vi "oscillograph (2).vi"() -> ()   [LabVIEW 2013]
panel:
  out "Fall time":string
  out "Rise time":string
  out "Period":string
  out "Vrms":string
  out "Vpp":string
  in  "Channels":T1(radio)
  in  "Exit":bool
  out "Waveform Graph":u8[](graph)
  in  "VISA Address":refnum<visa-resource-name>
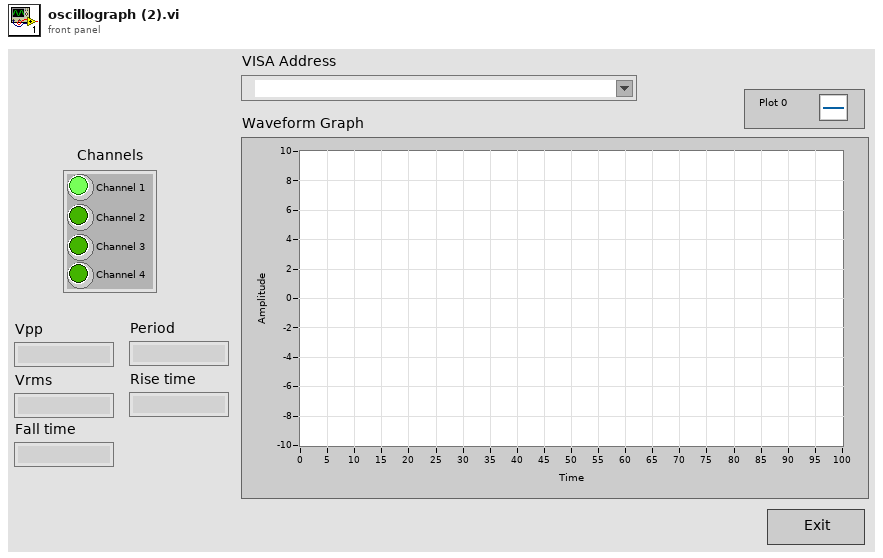
[diagram p1: front panel]
types:
  T1 = enum32{"Channel 1", "Channel 2", "Channel 3", "Channel 4"}
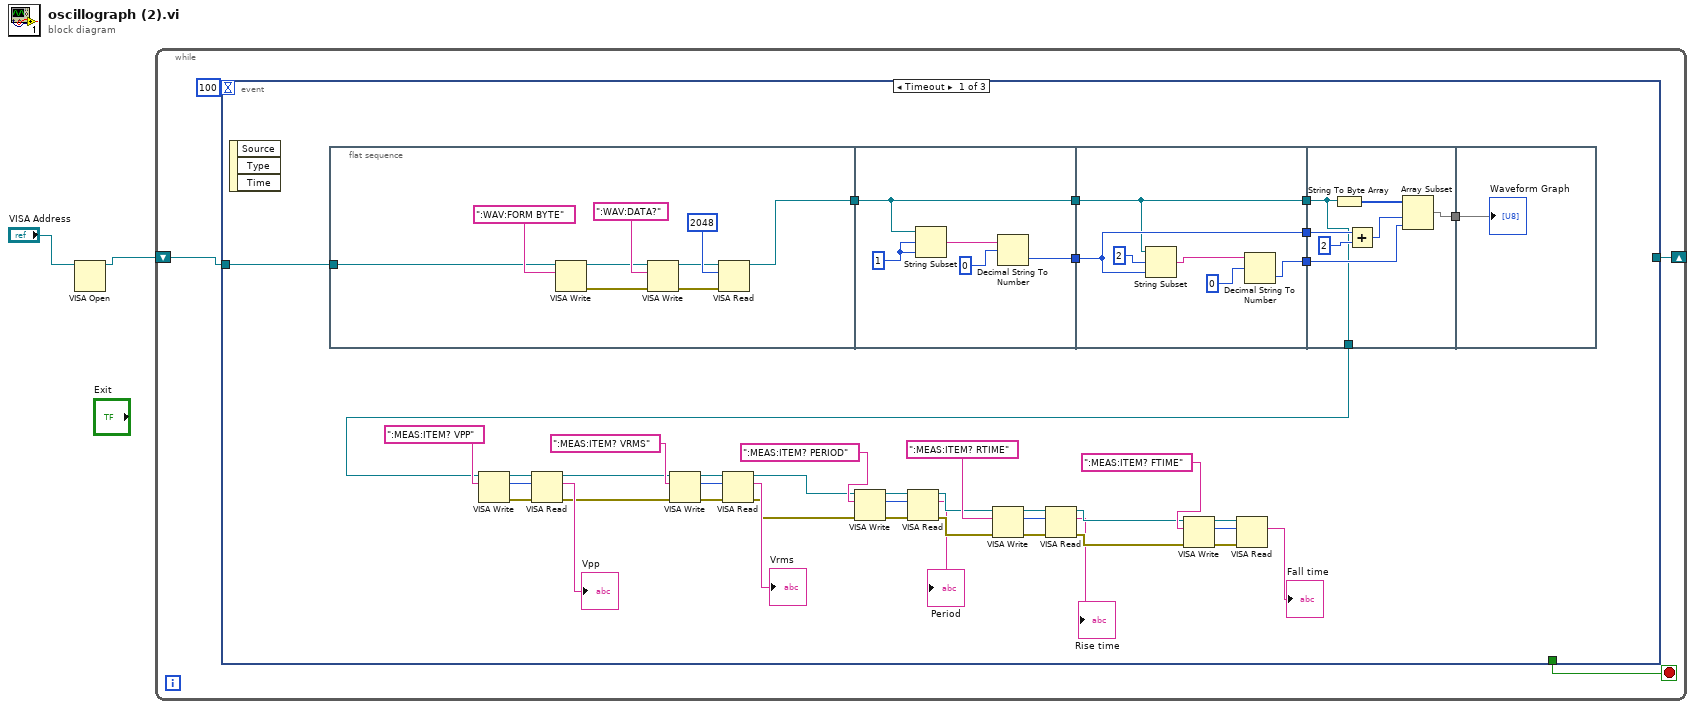
[diagram p0: block diagram]
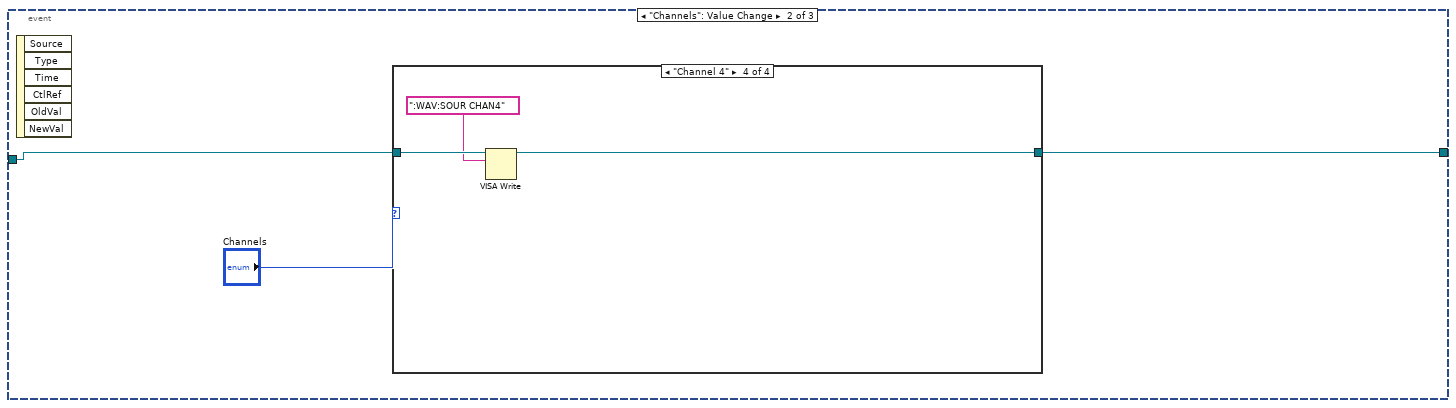
[diagram p2: hidden frame]
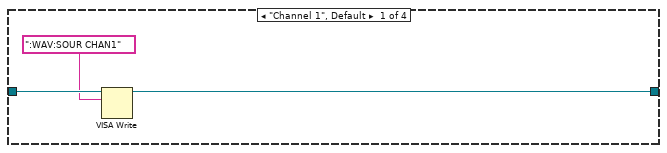
[diagram p3: hidden frame]
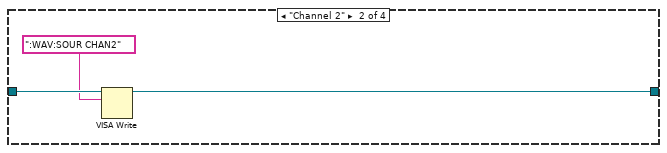
[diagram p4: hidden frame]
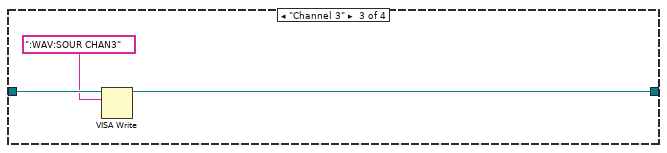
[diagram p5: hidden frame]
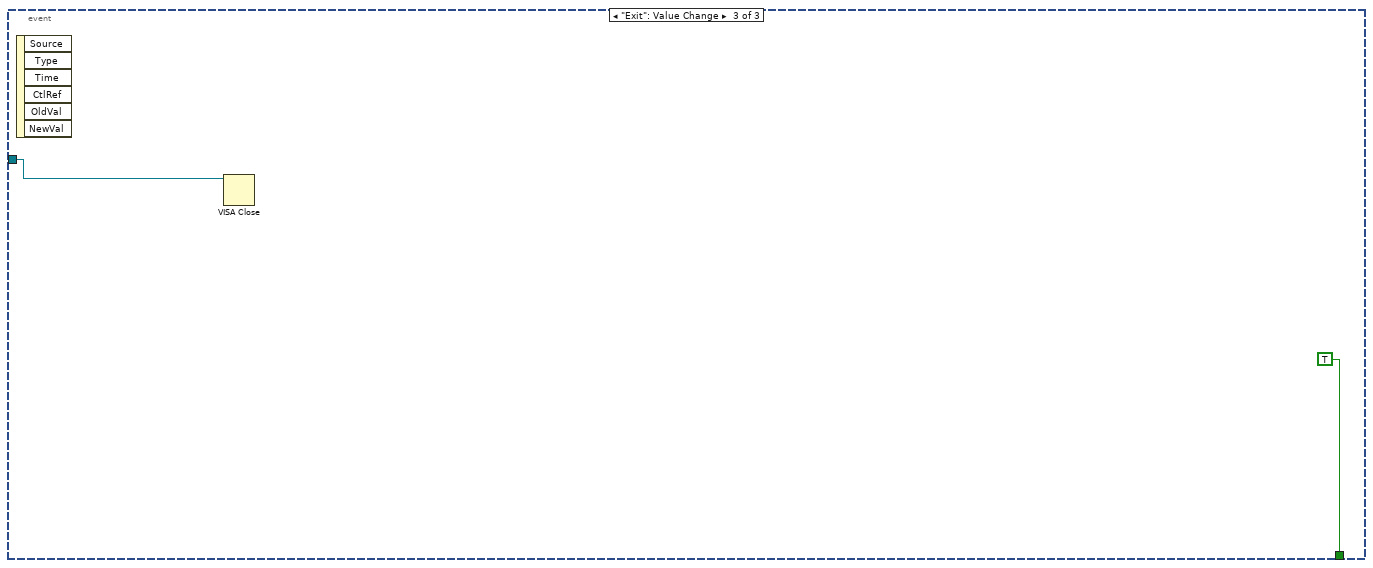
[diagram p6: hidden frame]
diagram:
  n1 = VISA Open(VISA resource name="VISA Address") -> (VISA resource name=w1:refnum<visa-resource-name>)  [unwired: 4 in, 1 out]
  n2 = while {
    shift-right: [w3] -> _
    shift-left: w1 -> [w5]
    stop <- w4 stop-if-true
    n3 = event shown="[0] Timeout" {
      selector: _ -> [_ _ _]
      dyn-events: _ -> [_ _ _]
      timeout: 100 -> [_ _ _]
      tunnel: w5 -> [w41 w78 w93]
      tunnel: [_ _ TRUE] -> w4
      tunnel: [_ w77 _] -> w3
      event Timeout {
        n4 = event-data() -> ()  [unwired: 1 in, 3 out]
        n5 = flat-sequence {
          tunnel: [w50] -> w48
          tunnel: w41 -> [w49]
          tunnel: w48 -> [w62]
          tunnel: [w62] -> w47
          tunnel: [w58] -> w46
          tunnel: w47 -> [w65]
          tunnel: w46 -> [w67]
          tunnel: [w67] -> w45
          tunnel: [w65] -> w44
          tunnel: [w63] -> w43
          tunnel: w45 -> [w75]
          tunnel: w44 -> [w69]
          tunnel: w43 -> [w73]
          tunnel: [w70] -> w42
          tunnel: [w69] -> w35
          tunnel: w42 -> [w76]
          frame #0 {
            n6 = VISA Write(VISA resource name=w49, write buffer=":WAV:FORM BYTE") -> (VISA resource name out=w51:refnum<visa-resource-name>, error out=w56:errorcluster)  [unwired: 1 in, 1 out]
            n7 = VISA Write(VISA resource name=w51, write buffer=":WAV:DATA?", error in (no error)=w56) -> (VISA resource name out=w52:refnum<visa-resource-name>, error out=w57:errorcluster)  [unwired: 1 out]
            n8 = VISA Read(VISA resource name=w52, byte count=u32 2048, error in (no error)=w57) -> (VISA resource name out=w50:refnum<visa-resource-name>)  [unwired: 3 out]
          }
          frame #1 {
            w61 = 1 ("offset (0)")
            n9 = String Subset(string=w62, offset (0)=w61, length (rest)=w61) -> (substring=w60:string)
            n10 = Decimal String To Number(string=w60, offset=0) -> (number=w58:i32)  [unwired: 1 in, 1 out]
          }
          frame #2 {
            n11 = String Subset(string=w65, offset (0)=2 ("index"), length (rest)=w67) -> (substring=w64:string)
            n12 = Decimal String To Number(string=w64, offset=0) -> (number=w63:i32)  [unwired: 1 in, 1 out]
          }
          frame #3 {
            n13 = String To Byte Array(string=w69) -> (unsigned byte array=w71:u8[])
            n14 = Add(x=w75, y=2) -> (x+y=w72:i32)
            n15 = Array Subset(array=w71, index=w72, length=w73) -> (w70:u8[])
          }
          frame #4 {
            "Waveform Graph" <- w76
          }
        }
        n16 = VISA Write(VISA resource name=w35, write buffer=":MEAS:ITEM? VPP") -> (VISA resource name out=w39:refnum<visa-resource-name>, return count=w37:u32, error out=w38:errorcluster)  [unwired: 1 in]
        n17 = VISA Read(VISA resource name=w39, byte count=w37, error in (no error)=w38) -> (VISA resource name out=w30:refnum<visa-resource-name>, read buffer=→"Vpp":string, error out=w29:errorcluster)  [unwired: 1 out]
        n18 = VISA Write(VISA resource name=w30, write buffer=":MEAS:ITEM? VRMS", error in (no error)=w29) -> (VISA resource name out=w34:refnum<visa-resource-name>, return count=w32:u32, error out=w33:errorcluster)
        n19 = VISA Read(VISA resource name=w34, byte count=w32, error in (no error)=w33) -> (VISA resource name out=w15:refnum<visa-resource-name>, read buffer=→"Vrms":string, error out=w12:errorcluster)  [unwired: 1 out]
        n20 = VISA Write(VISA resource name=w15, write buffer=":MEAS:ITEM? PERIOD", error in (no error)=w12) -> (VISA resource name out=w27:refnum<visa-resource-name>, return count=w25:u32, error out=w26:errorcluster)
        n21 = VISA Read(VISA resource name=w27, byte count=w25, error in (no error)=w26) -> (VISA resource name out=w14:refnum<visa-resource-name>, read buffer=→"Period":string, error out=w11:errorcluster)  [unwired: 1 out]
        n22 = VISA Write(VISA resource name=w14, write buffer=":MEAS:ITEM? RTIME", error in (no error)=w11) -> (VISA resource name out=w24:refnum<visa-resource-name>, return count=w22:u32, error out=w23:errorcluster)
        n23 = VISA Read(VISA resource name=w24, byte count=w22, error in (no error)=w23) -> (VISA resource name out=w13:refnum<visa-resource-name>, read buffer=→"Rise time":string, error out=w10:errorcluster)  [unwired: 1 out]
        n24 = VISA Write(VISA resource name=w13, write buffer=":MEAS:ITEM? FTIME", error in (no error)=w10) -> (VISA resource name out=w21:refnum<visa-resource-name>, return count=w19:u32, error out=w20:errorcluster)
        n25 = VISA Read(VISA resource name=w21, byte count=w19, error in (no error)=w20) -> (read buffer=→"Fall time":string)  [unwired: 3 out]
      }
      event "Channels": Value Change {
        n26 = event-data() -> ()  [unwired: 1 in, 6 out]
        n27 = case shown="\"Channel 4\"" "Channels" {
          tunnel: w78 -> [w82 w85 w88 w91]
          tunnel: [w80 w83 w86 w89] -> w77
          frame "Channel 1", Default {
            n28 = VISA Write(VISA resource name=w82, write buffer=":WAV:SOUR CHAN1") -> (VISA resource name out=w80:refnum<visa-resource-name>)  [unwired: 1 in, 2 out]
          }
          frame "Channel 2" {
            n29 = VISA Write(VISA resource name=w85, write buffer=":WAV:SOUR CHAN2") -> (VISA resource name out=w83:refnum<visa-resource-name>)  [unwired: 1 in, 2 out]
          }
          frame "Channel 3" {
            n30 = VISA Write(VISA resource name=w88, write buffer=":WAV:SOUR CHAN3") -> (VISA resource name out=w86:refnum<visa-resource-name>)  [unwired: 1 in, 2 out]
          }
          frame "Channel 4" {
            n31 = VISA Write(VISA resource name=w91, write buffer=":WAV:SOUR CHAN4") -> (VISA resource name out=w89:refnum<visa-resource-name>)  [unwired: 1 in, 2 out]
          }
        }
      }
      event "Exit": Value Change {
        n32 = event-data() -> ()  [unwired: 1 in, 6 out]
        n33 = VISA Close(VISA resource name=w93) -> ()  [unwired: 1 in, 1 out]
      }
    }
  }
